vi "CloseFile.vi"(0 "object in":refnum<class "ErrorLogFile.lvclass">, 5 "Error In":errorcluster) -> (14 "object out":refnum<class "ErrorLogFile.lvclass">, 19 "Error Out":errorcluster)   [LabVIEW 2019, in "ErrorLogFile.lvclass"]
uses:
  ErrorLogFile.lvclass
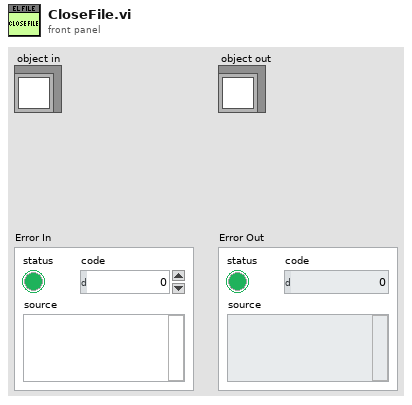
[diagram p1: front panel]
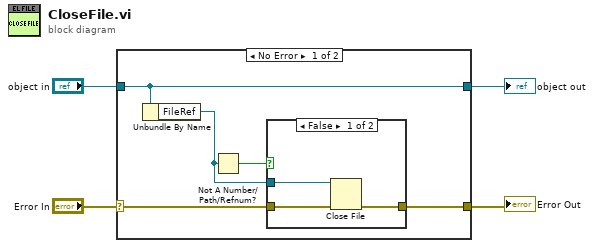
[diagram p0: block diagram]
diagram:
  n1 = case shown="No Error" "Error In" {
    selector: "Error In" -> [w6 w15]
    tunnel: [w5 w15] -> w3
    tunnel: [w9 w14] -> w1
    tunnel: "object in" -> [w9 w14]
    frame No Error {
      n2 = Unbundle By Name(w9) -> ("FileRef"=w7:refnum<file>)
      n3 = Not A Number/Path/Refnum?(number/path/refnum=w7) -> (NaN/Path/Refnum?=w8:bool)
      n4 = case shown="False" w8 {
        tunnel: w6 -> [w12 w13]
        tunnel: [w11 w13] -> w5
        tunnel: w7 -> [w10 _]
        frame False {
          n5 = Close File(refnum=w10, error in=w12) -> (error out=w11:errorcluster)  [unwired: 1 out]
        }
        frame True {
        }
      }
    }
    frame Error {
    }
  }
  "Error Out" <- w3
  "object out" <- w1
